vi "Insert_Menu.vi"(0 "menu reference":refnum<k9>, 5 "LEVEL1":string[](array[string])=["File", "Units"], 7 "SubMenu1":string[](array[string])=["Stop Execution", "Mode Demo"], 9 "SubMenu2":string[](array[string])=["mm", "inches"], 11 "error in (no error)":errorcluster) -> (4 "menu reference out":refnum<k9>, 15 "error out":errorcluster)   [LabVIEW 2024, in "Utilities.lvlib"]
uses:
  Utilities.lvlib
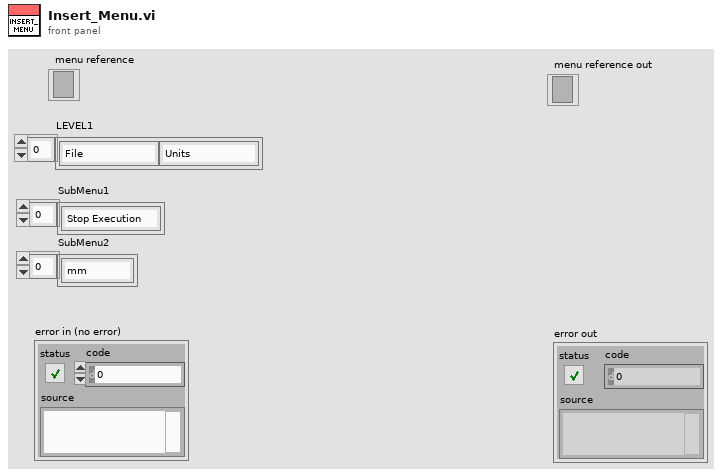
[diagram p1: front panel]
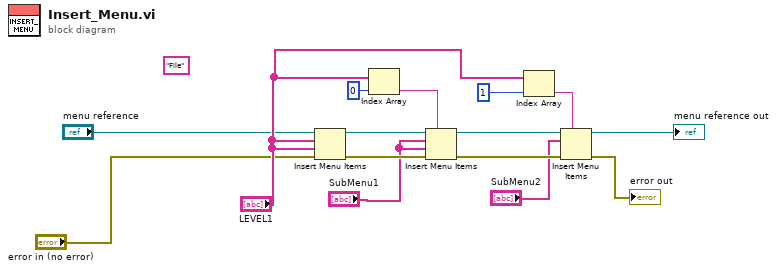
[diagram p0: block diagram]
diagram:
  (unwired) "File" ("menu tag")
  n1 = Insert Menu Items(6:"error in (no error)", 7:"LEVEL1", 8:"LEVEL1", 9:"menu reference") -> (0:w14:errorcluster, 3:w15:refnum<k9>)  [unwired: 2 in, 1 out]
  n2 = Index Array(array="LEVEL1", index=0) -> (element=w12:string)
  n3 = Insert Menu Items(5:w12, 6:w14, 7:"SubMenu1", 8:"SubMenu1", 9:w15) -> (0:w9:errorcluster, 3:w8:refnum<k9>)  [unwired: 1 in, 1 out]
  n4 = Index Array(array="LEVEL1", index=1) -> (element=w7:string)
  n5 = Insert Menu Items(5:w7, 6:w9, 8:"SubMenu2", 9:w8) -> (0:→"error out":errorcluster, 3:→"menu reference out":refnum<k9>)  [unwired: 2 in, 1 out]
